vi "Export Image.vi"(5 "Always Overwrite":bool, 6 "Hide Grid":bool, 7 "Path":path, 8 "error in (no error)":errorcluster, 9 "Target":enum32{"File", "Clipboard"}(ring), 10 "File Type":enum32{"BMP", "EPS", "EMF", "PICT"}(ring), 11 "MixedSignalGraph in":refnum<class "MixedSignalGraph.lvclass">) -> (0 "error out":errorcluster, 3 "MixedSignalGraph out":refnum<class "MixedSignalGraph.lvclass">)   [LabVIEW 2015, in "MixedSignalGraph.lvclass"]
doc: "Exports a simplified image of the graph to the clipboard or a file.\n\nQControl Class wrapper around the <b>MixedSignalGraph : Export Image Method</b>.\n<b> </b> <b> </b>\n©2016 Q Software Innovations, LLC (QSI)\nwritten by Quentin Alldredge\nproduced in LabVIEW 2015\n\nsupport@qsoftwareinnovations.com\nwww.qsoftwareinnovations.com\n\nAll rights reserved.\n\nRedistribution and use in source and binary forms, with or without modification, are permitted provided that the following conditions are met:\n\n * Redistributions of source code must retain the above copyright notice, this list of conditions and the following disclaimer.\n * Redistributions in binary form must reproduce the above copyright notice, this list of conditions and the following disclaimer in the documentation and/or other materials provided with the distribution.\n * Neither the name of Q Software Innovations, LLC. nor the names of its contributors may be used to endorse or promote products derived from this software without specific prior written permission.\n\nTHIS SOFTWARE IS PROVIDED BY THE COPYRIGHT HOLDERS AND CONTRIBUTORS \"AS IS\" AND ANY EXPRESS OR IMPLIED WARRANTIES, INCLUDING, BUT NOT LIMITED TO, THE IMPLIED WARRANTIES OF MERCHANTABILITY AND FITNESS FOR A PARTICULAR PURPOSE ARE DISCLAIMED. IN NO EVENT SHALL THE COPYRIGHT OWNER OR CONTRIBUTORS BE LIABLE FOR ANY DIRECT, INDIRECT, INCIDENTAL, SPECIAL, EXEMPLARY, OR CONSEQUENTIAL DAMAGES (INCLUDING, BUT NOT LIMITED TO, PROCUREMENT OF SUBSTITUTE GOODS OR SERVICES; LOSS OF USE, DATA, OR PROFITS; OR BUSINESS INTERRUPTION) HOWEVER CAUSED AND ON ANY THEORY OF LIABILITY, WHETHER IN CONTRACT, STRICT LIABILITY, OR TORT (INCLUDING NEGLIGENCE OR OTHERWISE) ARISING IN ANY WAY OUT OF THE USE OF THIS SOFTWARE, EVEN IF ADVISED OF THE POSSIBILITY OF SUCH DAMAGE."
uses:
  MixedSignalGraph.lvclass
  MixedSignalGraph.lvclass/MixedSignalGraph.ctl
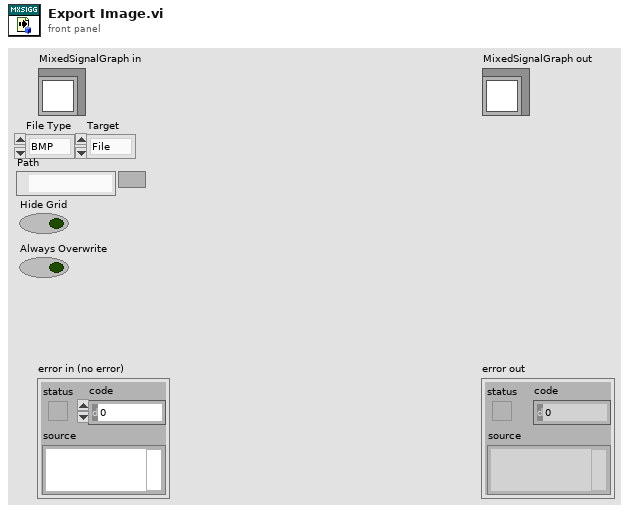
[diagram p1: front panel]
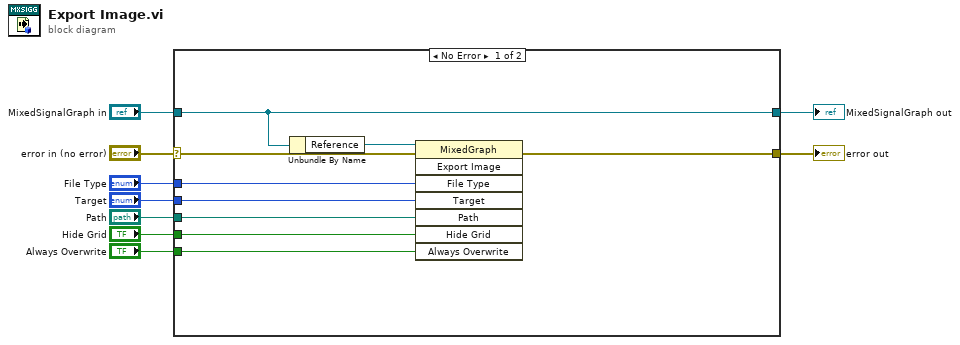
[diagram p0: block diagram]
diagram:
  n1 = case shown="No Error" "error in (no error)" {
    selector: "error in (no error)" -> [w18 w20]
    tunnel: [w17 w20] -> w8
    tunnel: [w16 w19] -> w6
    tunnel: "MixedSignalGraph in" -> [w16 w19]
    tunnel: "File Type" -> [w14 _]
    tunnel: "Target" -> [w13 _]
    tunnel: "Path" -> [w12 _]
    tunnel: "Hide Grid" -> [w11 _]
    tunnel: "Always Overwrite" -> [w10 _]
    frame No Error {
      n2 = Unbundle By Name(w16) -> ("Reference"=w15:refnum<vi>)
      n3 = invoke class="MixedGraph" method="Export Image"(reference=w15, error in=w18, "File Type"=w14, "Target"=w13, "Path"=w12, "Hide Grid"=w11, "Always Overwrite"=w10) -> (error out=w17:errorcluster)  [unwired: 1 in, 7 out]
    }
    frame Error {
    }
  }
  "error out" <- w8
  "MixedSignalGraph out" <- w6
